vi "Test Log Not Logging Error Message unless Error.vi"(8 "error in (no error)":errorcluster, 11 "Test Case In":refnum<class "Logger Test.lvclass">) -> (0 "error out":errorcluster, 3 "Test Case Out":refnum<class "Logger Test.lvclass">)   [LabVIEW 2020, in "Logger Test.lvclass"]
uses:
  Logger Test.lvclass
  Mock Log Handler/Mock Log Handler.lvclass
  Framework/Process/Process.lvclass
  Mock Process/Mock Process.lvclass
  Framework/Logging/Logging.lvclass
  C:/Users/anton/Documents/GitHub/Triarc-Framework/source/Framework/Process/Process.lvclass
  C:/Users/anton/Documents/GitHub/Triarc-Framework/source/Framework/Base/Base.lvclass
  C:/Users/anton/Documents/GitHub/Triarc-Framework/source/Framework/Error Handler Interface/Error Handler Interface.lvclass
  C:/Users/anton/Documents/GitHub/Triarc-Framework/source/Framework/Logging/Logging.lvclass
  C:/Users/anton/Documents/GitHub/Triarc-Framework/source/Framework Test/Mock Process/Mock Process.lvclass
  C:/Users/anton/Documents/GitHub/Triarc-Framework/source/Framework/Helper Loop/Helper Loop.lvclass
  <vilib>/Asteme/LUnit/Test Case.lvclass
  C:/Users/anton/Documents/GitHub/Triarc-Framework/source/Framework Test/Mock Log Handler/Mock Log Handler.lvclass
  C:/Program Files (x86)/National Instruments/LabVIEW 2020/vi.lib/Asteme/LUnit/Test Case.lvclass
  C:/Users/anton/Documents/GitHub/Triarc-Framework/source/Framework Test/Logger Test/Logger Test.lvclass
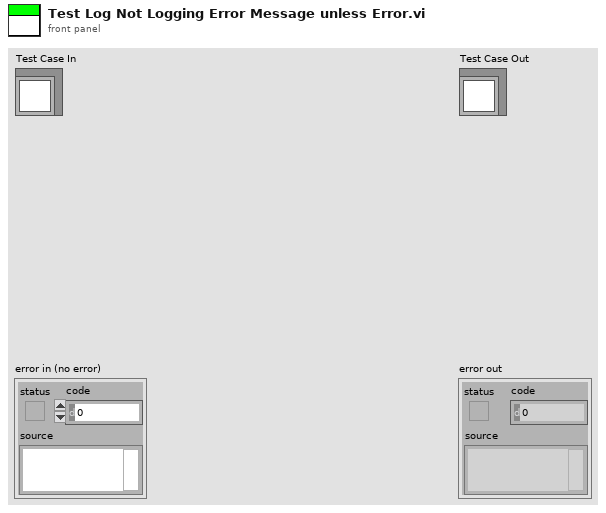
[diagram p1: front panel]
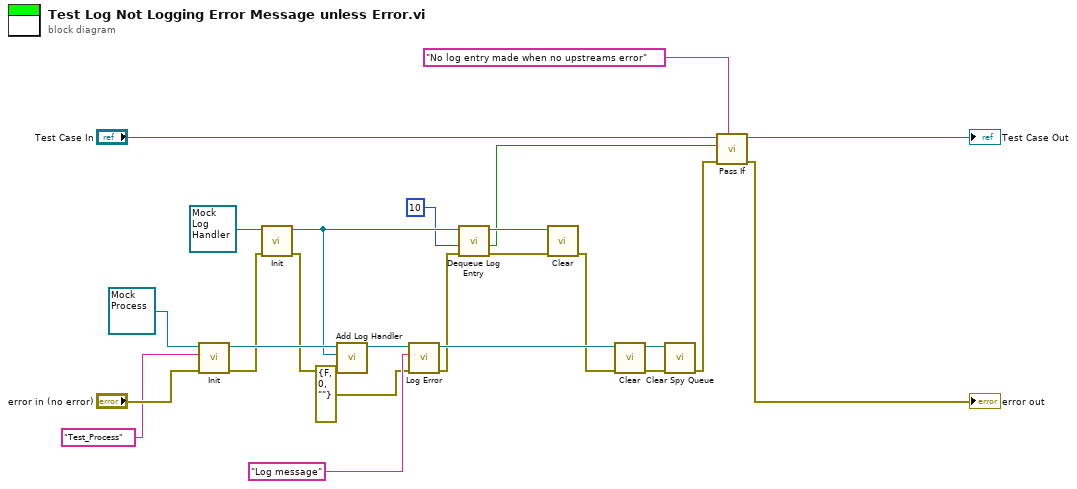
[diagram p0: block diagram]
diagram:
  n1 = call-dynamic "Init.vi"("error in (no error)"="error in (no error)", "Name"="Test_Process", "Mock Process In"=refnum<class "Mock Process.lvclass"> refnum) -> ("error out"=w16:errorcluster, "Mock Process Out"=w22:refnum<class "Mock Process.lvclass">)  [unwired: 7 in]
  n2 = call-dynamic "Init.vi"("error in (no error)"=w16, "Mock Log Handler In"=refnum<class "Mock Log Handler.lvclass"> refnum ("Mock Log Handler.lvclass")) -> ("error out"=w15:errorcluster, "Mock Log Handler Out"=w12:refnum<class "Mock Log Handler.lvclass">)  [unwired: 8 in]
  n3 = call "Add Log Handler.vi"("error in (no error)"=w15, "Log Handler"=w12, "Process in"=w22) -> ("Process out"=w10:refnum<class "Mock Process.lvclass">)  [unwired: 7 in, 1 out]
  n4 = call "Log Error.vi"("error in (no error)"=errorcluster {"status"=FALSE, "code"=0, "source"=""}, "Message"="Log message", "Logging In"=w10) -> ("error out"=w2:errorcluster, "Logging Out"=w9:refnum<class "Mock Process.lvclass">)  [unwired: 7 in]
  n5 = call "Dequeue Log Entry.vi"("error in (no error)"=w2, "timeout in ms (-1)"=10, "Mock Log Handler in"=w12) -> ("error out"=w13:errorcluster, "timed out?"=w1:bool, "Mock Log Handler out"=w14:refnum<class "Mock Log Handler.lvclass">)  [unwired: 5 in, 1 out]
  n6 = call-dynamic "Clear.vi"("error in (no error)"=w13, "Mock Log Handler In"=w14) -> ("error out"=w8:errorcluster)  [unwired: 8 in, 1 out]
  n7 = call-dynamic "Clear.vi"("error in (no error)"=w8, "Mock Process In"=w9) -> ("error out"=w20:errorcluster, "Mock Process Out"=w21:refnum<class "Mock Process.lvclass">)  [unwired: 8 in]
  n8 = call-dynamic "Clear Spy Queue.vi"("error in (no error)"=w20, "Mock Process In"=w21) -> ("error out"=w6:errorcluster)  [unwired: 8 in, 1 out]
  n9 = call <vilib>:"Pass If.vi"("Description"="No log entry made when no upstreams error", "error in (no error)"=w6, "Pass?"=w1, "Test Case In"="Test Case In") -> ("error out"=→"error out":errorcluster, "Test Case Out"=→"Test Case Out":refnum<class "Logger Test.lvclass">)  [unwired: 6 in]
